vi "TeddingtonClient.vi"() -> (0 "Time Of Value (s)":dbl format="%#.1f", 1 "Error":bool, 2 "Sea level Pressure String/mBar":dbl)   [LabVIEW 2010]
panel:
  out "Time Stamp GMT":timestamp
  out "data out":string
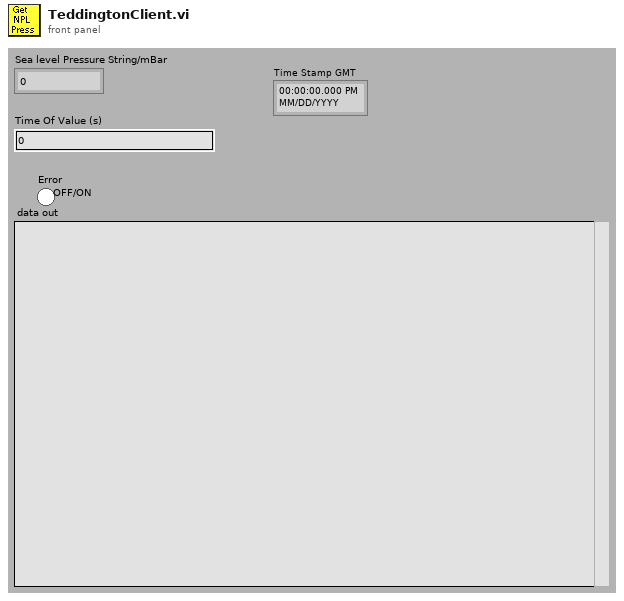
[diagram p1: front panel]
types:
  T1 = cluster{"second":i32, "minute":i32, "hour":i32, "day of month":i32, "month":i32, "year":i32, "day of week":i32, "day of year":i32, "is DST":i32}
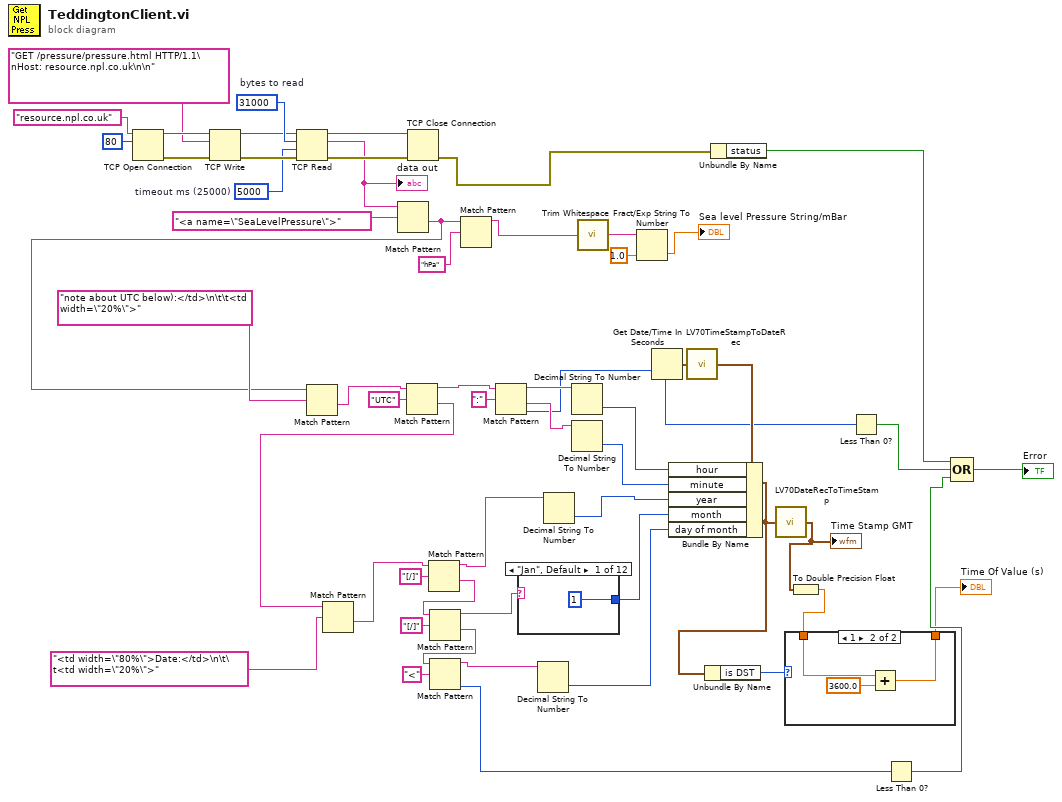
[diagram p0: block diagram]
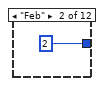
[diagram p3: hidden frame]
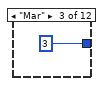
[diagram p4: hidden frame]
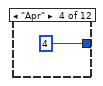
[diagram p5: hidden frame]
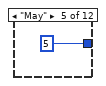
[diagram p6: hidden frame]
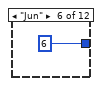
[diagram p7: hidden frame]
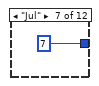
[diagram p8: hidden frame]
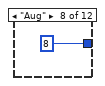
[diagram p9: hidden frame]
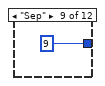
[diagram p10: hidden frame]
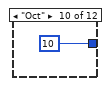
[diagram p11: hidden frame]
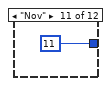
[diagram p12: hidden frame]
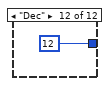
[diagram p13: hidden frame]
diagram:
  w3 = 5000  # timeout ms (25000)
  w48 = 31000  # bytes to read
  n1 = TCP Open Connection(address="resource.npl.co.uk", remote port or service name=u16 80 ("remote port")) -> (connection ID=w54:refnum<k5>, error out=w52:errorcluster)  [unwired: 1 in, 2 out]
  n2 = TCP Write(connection ID=w54, data in="GET /pressure/pressure.html HTTP/1.1\nHost: resource.npl.co.uk\n\n", error in (no error)=w52) -> (connection ID out=w47:refnum<k5>, error out=w51:errorcluster)  [unwired: 2 out]
  n3 = TCP Read(connection ID=w47, bytes to read=w48, error in (no error)=w51, 9:w3) -> (connection ID out=w50:refnum<k5>, data out=w5:string, error out=w49:errorcluster)  [unwired: 1 out]
  "data out" <- w5
  n4 = Match Pattern(string=w5, regular expression="<a name=\"SeaLevelPressure\">") -> (after substring=w6:string)  [unwired: 4 out]
  n5 = Match Pattern(string=w6, regular expression="note about UTC below):</td>\n\t\t<td width=\"20%\">") -> (after substring=w41:string)  [unwired: 4 out]
  n6 = Match Pattern(string=w41, regular expression="UTC") -> (before substring=w36:string, after substring=w22:string)  [unwired: 3 out]
  n7 = Match Pattern(string=w22, regular expression="<td width=\"80%\">Date:</td>\n\t\t<td width=\"20%\">") -> (after substring=w34:string)  [unwired: 4 out]
  n8 = TCP Close Connection(connection ID=w50, error in (no error)=w49) -> (error out=w9:errorcluster)  [unwired: 2 out]
  n9 = Match Pattern(string=w34, regular expression="[/]") -> (before substring=w30:string, after substring=w29:string)  [unwired: 3 out]
  n10 = Match Pattern(string=w29, regular expression="[/]") -> (before substring=w27:string, after substring=w28:string)  [unwired: 3 out]
  n11 = Match Pattern(string=w28, regular expression="<") -> (before substring=w25:string, offset past match=w16:i32)  [unwired: 3 out]
  n12 = Match Pattern(string=w6, regular expression="hPa") -> (before substring=w1:string)  [unwired: 4 out]
  n13 = Match Pattern(string=w36, regular expression=":") -> (before substring=w40:string, after substring=w39:string, offset past match=w15:i32)  [unwired: 2 out]
  n14 = case shown="\"Jan\", Default" w27 {
    tunnel: [1 ("month") 2 ("month") 3 ("month") 4 ("month") 5 ("month") 6 ("month") 7 ("month") 8 ("month") 9 ("month") 10 ("month") 11 ("month") 12 ("month")] -> w26
    frame "Jan", Default {
    }
    frame "Feb" {
    }
    frame "Mar" {
    }
    frame "Apr" {
    }
    frame "May" {
    }
    frame "Jun" {
    }
    frame "Jul" {
    }
    frame "Aug" {
    }
    frame "Sep" {
    }
    frame "Oct" {
    }
    frame "Nov" {
    }
    frame "Dec" {
    }
  }
  n15 = Decimal String To Number(string=w25) -> (number=w24:i32)  [unwired: 3 out]
  n16 = Decimal String To Number(string=w30) -> (number=w31:i32)  [unwired: 3 out]
  n17 = Decimal String To Number(string=w40) -> (number=w37:i32)  [unwired: 3 out]
  n18 = Decimal String To Number(string=w39) -> (number=w38:i32)  [unwired: 3 out]
  n19 = call <vilib>:"Trim Whitespace.vi"("string"=w1) -> ("trimmed string"=w12:string)  [unwired: 1 in]
  n20 = Fract/Exp String To Number(string=w12, default (0 dbl)=1.0 ("default (0 DBL)")) -> (number=→"Sea level Pressure String/mBar":dbl)  [unwired: 3 out]
  n21 = Get Date/Time In Seconds() -> (seconds since 1Jan1904=w2:timestamp)
  n22 = call <vilib>:"LV70TimeStampToDateRec.vi"("time stamp"=w2) -> ("date time rec"=w21:T1)
  n23 = Bundle By Name(cluster=w21, "hour"=w37, "minute"=w38, "year"=w31, "month"=w26, "day of month"=w24) -> (w19:T1)
  n24 = Unbundle By Name(w19) -> ("is DST"=w18:i32)
  n25 = Unbundle By Name(w9) -> ("status"=w8:bool)
  n26 = call <vilib>:"LV70DateRecToTimeStamp.vi"("date time rec"=w19) -> ("Time Stamp"=w20:timestamp)
  "Time Stamp GMT" <- w20
  n27 = To Double Precision Float(number=w20) -> (double precision float=w17:dbl)
  n28 = case shown="1" w18 {
    tunnel: w17 -> [w69 w72]
    tunnel: [w69 w70] -> w4
    frame 0, Default {
    }
    frame 1 {
      n29 = Add(x=w72, y=3600.0) -> (x+y=w70:dbl)
    }
  }
  "Time Of Value (s)" <- w4
  n30 = Less Than 0?(x=w15) -> (x < 0?=w10:bool)
  n31 = Less Than 0?(x=w16) -> (x < 0?=w11:bool)
  n32 = Compound Arithmetic op=OR(w8, w10, w11) -> (→"Error":bool)
